vi "Create NT Scalar.vi"(8 "error in":errorcluster, 9 "value fields":T1, 10 "type code":T2=enum."AnyA") -> (0 "error out":errorcluster, 3 "PV Data out":refnum<class "PV Data.lvclass">)   [LabVIEW 2020, in "PV Access.lvlib" / "PV Data.lvlib" / "PV Data.lvclass"]
uses:
  PV Data.lvclass
  PV Access.lvlib
  Type Code.ctl
  PV Data.lvlib
  Value Fields.ctl
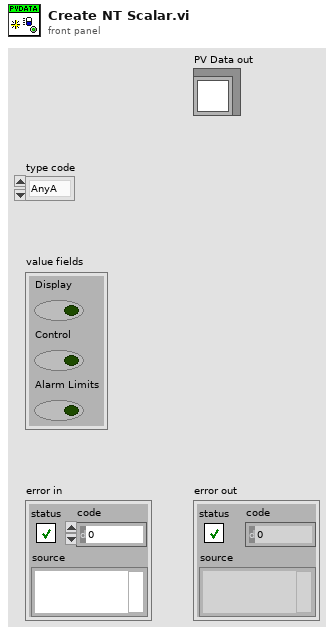
[diagram p1: front panel]
types:
  T1 = typedef "PV Access.lvlib/PV Data.lvlib/Value Fields.ctl" = cluster{"Display":bool, "Control":bool, "Alarm Limits":bool}
  T2 = typedef "PV Access.lvlib/PV Data.lvlib/Type Code.ctl" = enum8{"Null", "Bool", "BoolA", "Int8", "Int8A", "Int16", "Int16A", "Int32", "Int32A", "Int64", "Int64A", "UInt8", "UInt8A", "UInt16", "UInt16A", "UInt32", "UInt32A", "UInt64", "UInt64A", "Float32", "Float32A", "Float64", "Float64A", "String", "StringA", "Struct", "StructA", "Union", "UnionA", "Any", "AnyA"}
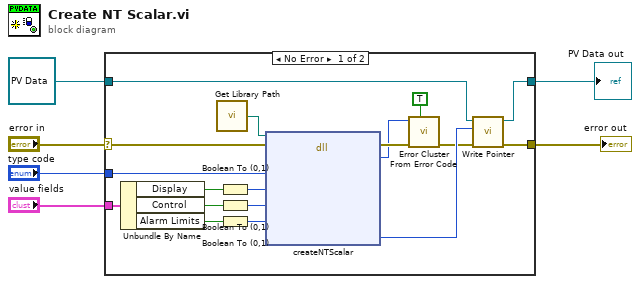
[diagram p0: block diagram]
diagram:
  n1 = case shown="No Error" "error in" {
    selector: "error in" -> [w24 w26]
    tunnel: [w8 w26] -> w6
    tunnel: "type code" -> [w20 _]
    tunnel: refnum<class "PV Data.lvclass"> refnum ("PV Data in") -> [w10 w25]
    tunnel: [w9 w25] -> w2
    tunnel: "value fields" -> [w18 _]
    frame No Error {
      n2 = Unbundle By Name(w18) -> ("Display"=w12:bool, "Control"=w15:bool, "Alarm Limits"=w17:bool)
      n3 = call "Get Library Path.vi"() -> ("Path"=w19:path)  [unwired: 1 in]
      n4 = Boolean To (0,1)(Boolean=w12) -> (0, 1=w13:i16)
      n5 = Boolean To (0,1)(Boolean=w15) -> (0, 1=w14:i16)
      n6 = Boolean To (0,1)(Boolean=w17) -> (0, 1=w16:i16)
      n7 = dll-call lib="?" fn="createNTScalar" ("createNT Scalar")(path in=w19, error in=w24, "type_code"=w20, "display"=w13, "control"=w14, "value_alarm"=w16) -> (error out=w22:errorcluster, "err_code"=w21:i32, "value"=w11:i64)  [unwired: 6 in, 1 out]
      n8 = call <vilib>:"Error Cluster From Error Code.vi"("show call chain? (False)"=TRUE, "error in (no error)"=w22, "error code (0)"=w21) -> ("error out"=w7:errorcluster)  [unwired: 6 in]
      n9 = call-dynamic "Write Pointer.vi"("error in (no error)"=w7, "Pointer"=w11, "Pointer Base in"=w10) -> ("error out"=w8:errorcluster, "Pointer Base out"=w9:refnum<class "PV Data.lvclass">)  [unwired: 7 in]
    }
    frame Error {
    }
  }
  "error out" <- w6
  "PV Data out" <- w2
